vi "Noise Cancel.vi"(7 "Filter config":T1={"Lower Cut-Off"=100.0, "Upper Cut-Off"=400.0}, 9 "Config":T3={"Active Index"=1, "Ref Index"=2, "Gain"=1.1, "Channel name"="Mic Diff", "Enable"=FALSE, "Offset"=0.0}, 11 "array":waveform(dbl)[](array[waveform])) -> (1 "Channel names":T2, 2 "Noise estimate (mVrms)":dbl format="%0.2f", 3 "waveform out":waveform(dbl))   [LabVIEW 2019]
doc: "This example demonstrates how to acquire a continuous amount of data (Waveform) using the DAQ device's internal clock. It also shows how to synchronize two devices for different device families (E Series, S Series, M Series, X Series, DSA, and SC Express), to simultaneously acquire the data.\n\nFor instructions on how to connect your signals to the DAQ device, refer to your device documentation."
uses:
  <vilib>/Analysis/NI_AALPro.lvlib
panel:
  # "Noise Cancellation"
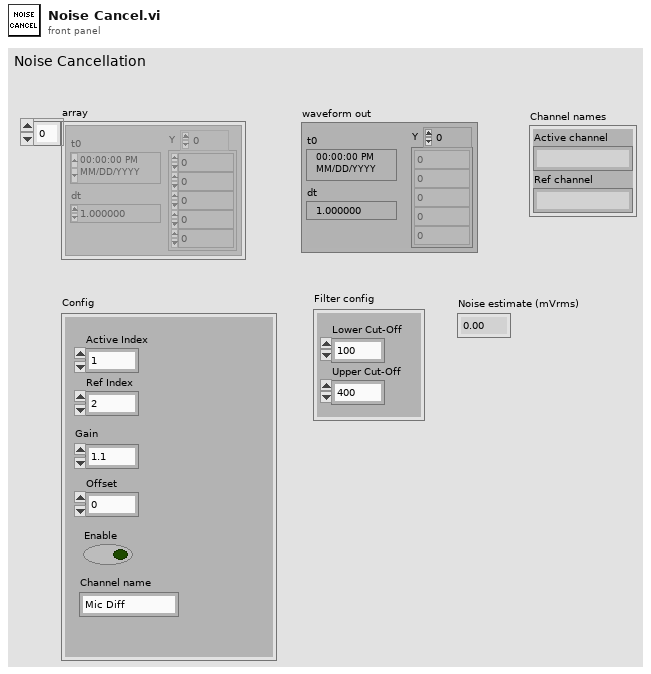
[diagram p1: front panel]
types:
  T1 = cluster{"Lower Cut-Off":dbl, "Upper Cut-Off":dbl}
  T2 = cluster{"Active channel":string, "Ref channel":string}
  T3 = cluster{"Active Index":i32, "Ref Index":i32, "Gain":dbl, "Channel name":string, "Enable":bool, "Offset":dbl}
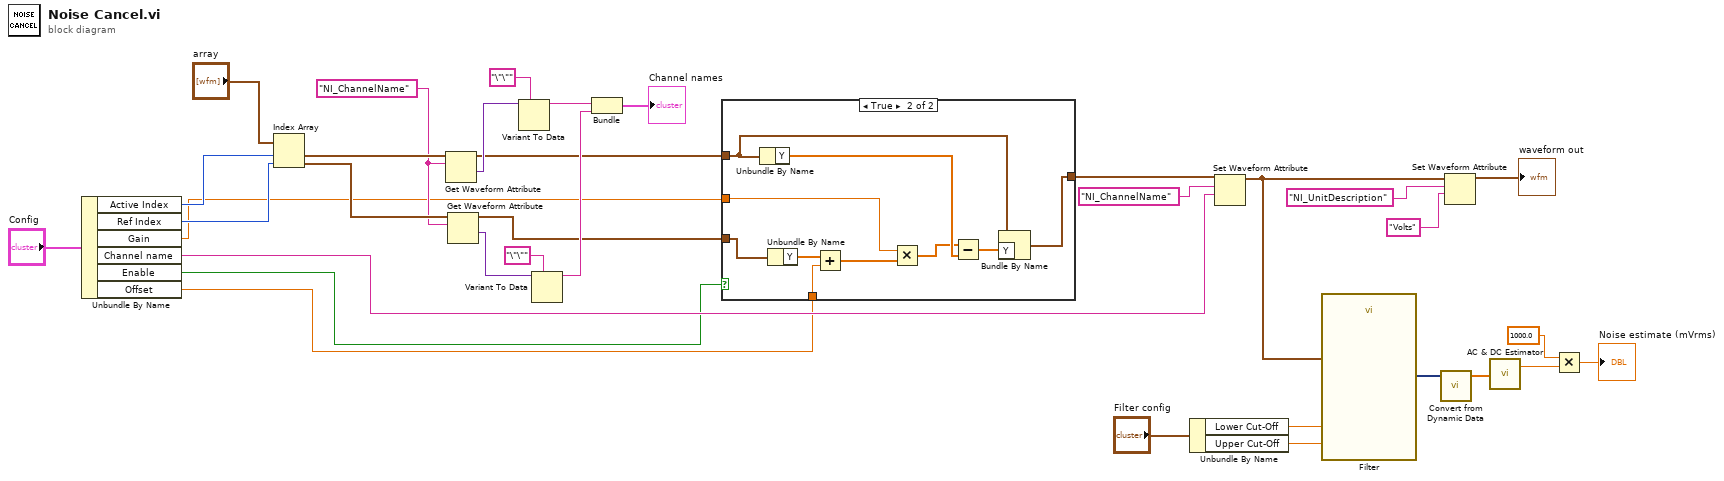
[diagram p0: block diagram]
diagram:
  w28 = "NI_ChannelName" ("name")
  n1 = Unbundle By Name("Config") -> ("Active Index"=w23:i32, "Ref Index"=w22:i32, "Gain"=w14:dbl, "Channel name"=w21:string, "Enable"=w11:bool, "Offset"=w10:dbl)
  n2 = Index Array(array="array", index #1=w23, index #2=w22) -> (element #1=w30:waveform(dbl), element #2=w29:waveform(dbl))
  n3 = Get Waveform Attribute(6:w28, 7:w30) -> (1:w19:variant, 3:w12:waveform(dbl))  [unwired: 2 in, 2 out]
  n4 = Get Waveform Attribute(6:w28, 7:w29) -> (1:w25:variant, 3:w15:waveform(dbl))  [unwired: 2 in, 2 out]
  n5 = Variant To Data(type="\"\"" ("name"), Variant=w19) -> (data=w18:string)  [unwired: 1 in, 1 out]
  n6 = Variant To Data(type="\"\"" ("name"), Variant=w25) -> (data=w16:string)  [unwired: 1 in, 1 out]
  n7 = Bundle("name"=w18, "name"=w16) -> (→"Channel names":cluster{"name":string, "name":string})  [unwired: 1 in]
  n8 = case shown="True" w11 {
    tunnel: w15 -> [_ w44]
    tunnel: w14 -> [_ w45]
    tunnel: [w35 w39] -> w13
    tunnel: w12 -> [w35 w36]
    tunnel: w10 -> [_ w41]
    frame False {
    }
    frame True {
      n9 = Unbundle By Name(w36) -> ("Y"=w38:dbl[])
      n10 = Unbundle By Name(w44) -> ("Y"=w43:dbl[])
      n11 = Add(x=w43, y=w41) -> (x+y=w42:dbl[])
      n12 = Multiply(x=w45, y=w42) -> (x*y=w37:dbl[])
      n13 = Subtract(x=w37, y=w38) -> (x-y=w40:dbl[])
      n14 = Bundle By Name(cluster=w36, "Y"=w40) -> (w39:waveform(dbl))
    }
  }
  n15 = Unbundle By Name("Filter config") -> ("Lower Cut-Off"=w5:dbl, "Upper Cut-Off"=w4:dbl)
  n16 = Set Waveform Attribute(5:w21, 6:"NI_ChannelName" ("name"), 7:w13) -> (3:w9:waveform(dbl))  [unwired: 1 in, 2 out]
  n17 = call "Filter"("Lower Cut-Off"=w5, "Upper Cut-Off"=w4, "Signal"=w9) -> ("Filtered Signal"=w8:dynamicdata)  [unwired: 7 in, 1 out]
  n18 = call "Convert from Dynamic Data"("Dynamic Data Type"=w8) -> ("Array"=w7:dbl[])  [unwired: 3 in]
  n19 = Set Waveform Attribute(5:"Volts" ("name"), 6:"NI_UnitDescription" ("name"), 7:w9) -> (3:→"waveform out":waveform(dbl))  [unwired: 1 in, 2 out]
  n20 = call <vilib>:"AC & DC Estimator.vi"("Signal (V)"=w7) -> ("AC estimate (Vrms)"=w3:dbl)  [unwired: 1 out]
  n21 = Multiply(x=1000.0, y=w3) -> (x*y=→"Noise estimate (mVrms)":dbl)
